vi "ErrHdlng.VI"(1 "ErrReporting":i32(ring) items=["DONTPRINT", "PRINTWARNINGS", "PRINTFATAL", "PRINTALL"]) -> (0 "ErrCode":i32)   [LabVIEW 2019, in "DAQ_Engine.lvclass"]
doc: "Developed by Kevin Thompson\nkevin@thompsonengineering.net\n\nCopyright 2020\nThompson Engineering, LLC\nSets the error handling for all subsequent function calls."
uses:
  DAQ_Engine.lvclass
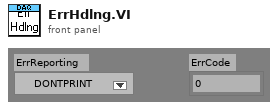
[diagram p1: front panel]
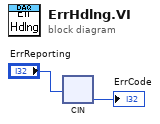
[diagram p0: block diagram]
diagram:
  n1 = cin("ErrReporting") -> (→"ErrCode":i32)  [unwired: 2 in]
